vi "CMI Sync V3 Set Channel 2 Pulse Count.vi"(8 "error in":errorcluster, 10 "Pulse count (0: infinite)":i32, 11 "session in":T1={"VISA"="", "baud rate [bd/s]"=115200, "source"=enum."Auto", "hv range"=enum."1kV", "fsrc is fixed"=FALSE, "fsrc [Hz]"=10000000.0, "freq integ [s]"=1.0, "freq filter"=5, "trig level"=enum."TTL 5V", "chn1 mode"=enum."Source divider", "chn1 level"=enum."Positive 5V", "chn2 mode"=enum."Source divider", "chn2 level"=enum."Positive 5V", "chn2 div"=1, "chn3 mode"=enum."Chn 1 Active", "chn3 level"=enum."Positive 5V"} {"chn2 div" min=1 max=100000000 step=1; "fsrc [Hz]" format="%_8p"}) -> (0 "error out":errorcluster, 3 "session out":T1={"VISA"="", "baud rate [bd/s]"=115200, "source"=enum."Auto", "hv range"=enum."1kV", "fsrc is fixed"=FALSE, "fsrc [Hz]"=10000000.0, "freq integ [s]"=1.0, "freq filter"=5, "trig level"=enum."TTL 5V", "chn1 mode"=enum."Source divider", "chn1 level"=enum."Positive 5V", "chn2 mode"=enum."Source divider", "chn2 level"=enum."Positive 5V", "chn2 div"=1, "chn3 mode"=enum."Chn 1 Active", "chn3 level"=enum."Positive 5V"} {"chn2 div" min=1 max=100000000 step=1; "fsrc [Hz]" format="%_8p"})   [LabVIEW 2020, in "AWG.lvlib" / "CMI Sync Unit V3.lvlib"]
doc: "Sets pulse count of channel 2. Use zero to infinite pulse train."
uses:
  CMI Sync Unit V3.lvlib
  CMI Sync V3 session.ctl
  CMI Sync V3 Reference Clock Source.ctl
  CMI Sync V3 HV input Range.ctl
  CMI Sync V3 Trigger Input Level.ctl
  CMI Sync V3 Channel 1 Mode.ctl
  CMI Sync V3 Channel Output Levels.ctl
  CMI Sync V3 Channel 2 Mode.ctl
  CMI Sync V3 Channel 3 Mode.ctl
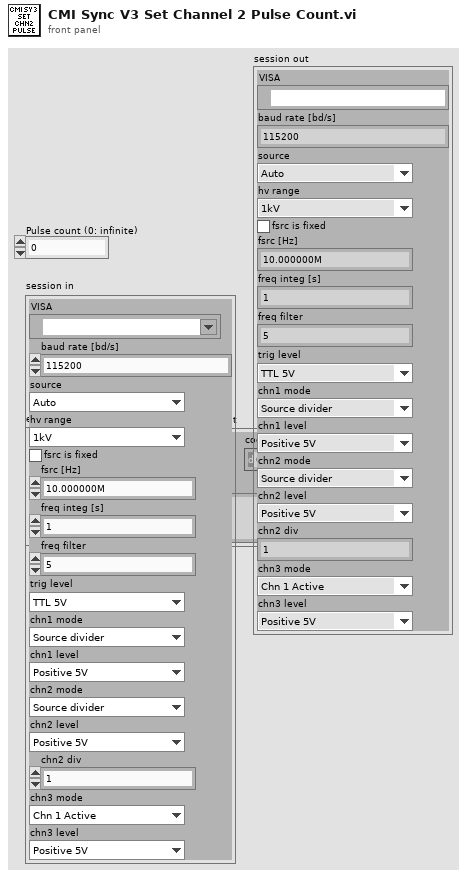
[diagram p1: front panel]
types:
  T1 = typedef "AWG.lvlib/CMI Sync Unit V3.lvlib/CMI Sync V3 session.ctl" = cluster{"VISA":refnum<visa-resource-name>, "baud rate [bd/s]":i32, "source":T2, "hv range":T3, "fsrc is fixed":bool, "fsrc [Hz]":dbl, "freq integ [s]":dbl, "freq filter":i32, "trig level":T4, "chn1 mode":T5, "chn1 level":T6, "chn2 mode":T7, "chn2 level":T6, "chn2 div":i32, "chn3 mode":T8, "chn3 level":T6}
  T2 = typedef "AWG.lvlib/CMI Sync Unit V3.lvlib/CMI Sync V3 Reference Clock Source.ctl" = enum16{"Auto", "Internal", "Logic", "Sine", "HV"}
  T3 = typedef "AWG.lvlib/CMI Sync Unit V3.lvlib/CMI Sync V3 HV input Range.ctl" = enum16{"10V", "60V", "250V", "1kV"}
  T4 = typedef "AWG.lvlib/CMI Sync Unit V3.lvlib/CMI Sync V3 Trigger Input Level.ctl" = enum16{"LVCMOS 3V3", "TTL 5V"}
  T5 = typedef "AWG.lvlib/CMI Sync Unit V3.lvlib/CMI Sync V3 Channel 1 Mode.ctl" = enum16{"Source divider", "DDS absolute", "DDS ratio", "DDS ratio M/N"}
  T6 = typedef "AWG.lvlib/CMI Sync Unit V3.lvlib/CMI Sync V3 Channel Output Levels.ctl" = enum16{"Positive 3V3", "Negative 3V3", "Positive 5V", "Negative 5V"}
  T7 = typedef "AWG.lvlib/CMI Sync Unit V3.lvlib/CMI Sync V3 Channel 2 Mode.ctl" = enum16{"Source divider", "Chn 1 divide"}
  T8 = typedef "AWG.lvlib/CMI Sync Unit V3.lvlib/CMI Sync V3 Channel 3 Mode.ctl" = enum16{"Chn 1 Active", "Chn 2 Active", "Chn 1 Trigger", "Chn 2 Trigger", "Gate", "PPS", "10MHz"}
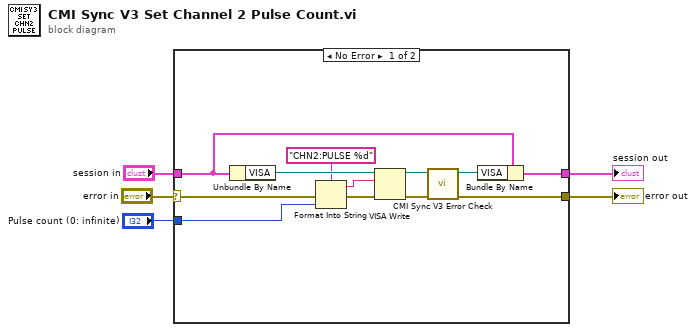
[diagram p0: block diagram]
diagram:
  n1 = case shown="No Error" "error in" {
    selector: "error in" -> [w10 w19]
    tunnel: "session in" -> [w17 w18]
    tunnel: [w16 w18] -> w2
    tunnel: [w11 w19] -> w3
    tunnel: "Pulse count (0: infinite)" -> [w6 _]
    frame No Error {
      n2 = Unbundle By Name(w17) -> ("VISA"=w15:refnum<visa-resource-name>)
      n3 = Format Into String(format string="CHN2:PULSE %d", error in=w10, w6) -> (resulting string=w8:string, error out=w9:errorcluster)  [unwired: 1 in]
      n4 = VISA Write(VISA resource name=w15, write buffer=w8, error in (no error)=w9) -> (VISA resource name out=w13:refnum<visa-resource-name>, error out=w14:errorcluster)  [unwired: 1 out]
      n5 = call "CMI Sync V3 Error Check.vi"("error in"=w14, "VISA in"=w13) -> ("error out"=w11:errorcluster, "VISA out"=w12:refnum<visa-resource-name>)  [unwired: 7 in, 1 out]
      n6 = Bundle By Name(cluster=w17, "VISA"=w12) -> (w16:T1)
    }
    frame Error {
    }
  }
  "error out" <- w3
  "session out" <- w2
